vi "Measurement.vi"(8 "error in (no error)":errorcluster, 9 "Grandeza":string, 10 "Multiplicador":dbl, 11 "Multimeter in":refnum<class "Multimeter.lvclass">) -> (0 "error out":errorcluster, 2 "Measurement":dbl, 3 "Multimeter out":refnum<class "Multimeter.lvclass">)   [LabVIEW 2015, in "Multimeter.lvclass"]
doc: "VI used to measure Value using the multimeter"
uses:
  Multimeter.lvclass
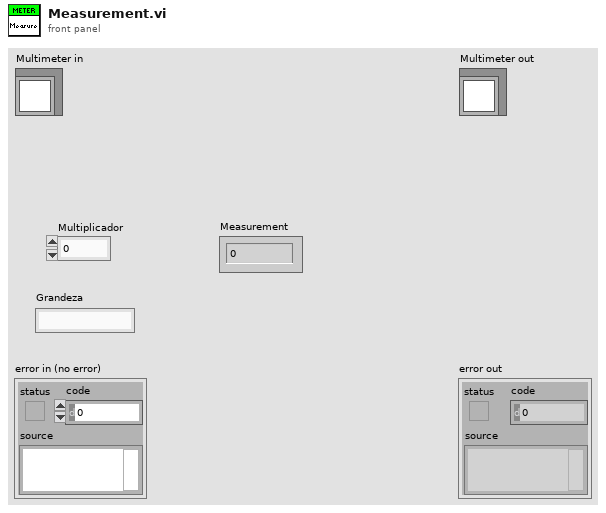
[diagram p1: front panel]
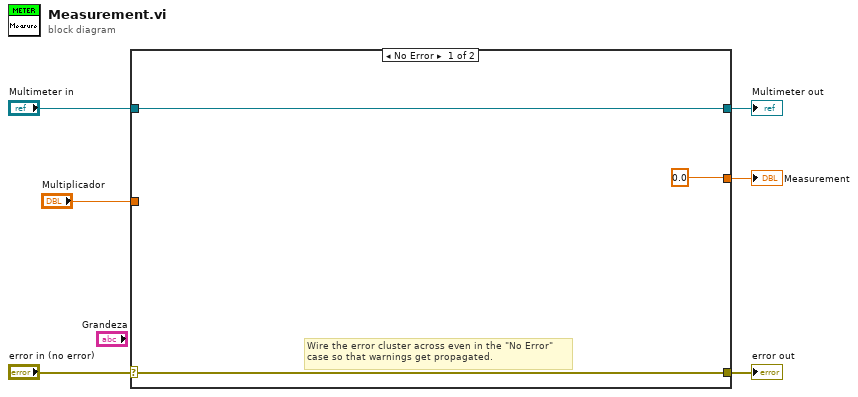
[diagram p0: block diagram]
diagram:
  n1 = case shown="No Error" "error in (no error)" {
    selector: "error in (no error)" -> [w8 w11]
    tunnel: [w8 w11] -> w5
    tunnel: [w9 w10] -> w3
    tunnel: "Multimeter in" -> [w9 w10]
    tunnel: [0.0 _] -> w2
    tunnel: "Multiplicador" -> [_ _]
    frame No Error {
      # "Wire the error cluster across even in the \"No Error\"\ncase so that warnings get propagated."
    }
    frame Error {
    }
  }
  "error out" <- w5
  "Multimeter out" <- w3
  "Measurement" <- w2
